vi "Robot Global Data.vi"() -> ()   [LabVIEW 2011]
doc: "This global VI can contain as many global variables as you need. Place a control on the panel, give it a good name. To read or write to it from a VI, drag the icon to the diagram of that VI. You can also drag from the project. Click on the node to change which global you access. You shouldn't have multiple locations writing to a global or it will cause a race-condition."
uses:
  <vilib>/Rock Robotics/WPI/Camera/WPI_CameraImageSize.ctl
  <vilib>/Rock Robotics/WPI/Camera/WPI_CameraWhite Balance Values.ctl
  <vilib>/Rock Robotics/WPI/Camera/WPI_CameraExposure Values.ctl
panel:
  out "Right Drive Distance":dbl
  in  "Binary Path":path
  in  "Harvester Speed":dbl=0.8
  out "Shoot":bool
  out "Shooter Primed":bool
  in  "Right Limit":dbl=3.55
  in  "Left Limit":dbl=1.45
  out "Dashboard DI 2":bool
  out "Record Iteration":dbl
  in  "Shooter Array":dbl[][](array[numeric])
  out "Ball S3 Process":bool
  out "Ball S12 Process":bool
  out "SP 3 Triggered":bool
  out "Conveyer Output":dbl
  out "Harvester Output":dbl
  out "Balls in Robot":dbl
  out "SP 2 Triggered":bool
  out "SP 1 Triggered":bool
  out "Ramp Actuator Output":dbl
  in  "RA Up Volt":dbl=3.7
  in  "RA Down Volt":dbl=1.55
  out "Ramp Actuator Case":dbl
  out "Ramp Actuator Activated":bool
  out "Gyro_Rate":dbl
  in  "Home Position":dbl=2.5
  out "REncoderRate":dbl
  out "LEncoderRate":dbl
  out "Manual Overide":bool
  out "Shooter Output":dbl
  out "Distance To Target":dbl
  out "Home Button":bool
  out "Turret Case":dbl
  out "Lock On Lights":dbl
  out "Raw Turret":dbl
  in  "Enable Color":bool
  in  "Brightness":dbl=30.0
  in  "Exposure":T1=enum."Flicker-free 60 Hz"
  in  "White Balance":T2=enum."Fixed fluorescent 1"
  out "file_read_test_5":dbl
  out "file_read_test_4":dbl
  out "file_read_test_3":dbl
  out "file_read_test_2":dbl
  out "file_read_test_1":dbl
  in  "GlobalVariableArray 2":cluster{"name":string, "va;":dbl}[](array[cluster])=[{"name"="Val1", "va;"=1.0}, {"name"="Val2", "va;"=2.0}, {"name"="Val3", "va;"=3.0}, {"name"="Val4", "va;"=4.0}]
  out "YStart":dbl
  out "XStart":dbl
  in  "Auton Files":string[](array[string])
  in  "Current Auton File":string
  out "Number of Auton Files":dbl
  out "Auton Distance Traveled":dbl
  out "Auton Index":sgl
  out "Robot Angle":dbl
  out "Left Drive Distance":dbl
  in  "Auton Array":dbl[][](array[numeric])
  out "Target Array":T3(array[cluster])
  out "Turret Rotation":dbl
  in  "Camera Settings":T5={"fps"=15, "compression"=30, "Image Size"=enum."320x240"}
  in  "RightShifter_Pos":dbl=0.25
  in  "LeftShifter_Pos":dbl=0.75
  out "Dashboard DI 4":bool
  out "Right Drive Output":dbl
  out "Left Drive Output":dbl
  in  "Camera Address":string="10.0.27.11"
  in  "LED toggle rate (ms)":u32=20
  in  "Enable Vision":bool=TRUE
  # "Sensor Feedback"
  # "Auton and Shooter CSV info"
  # "Motor Outputs"
  # "Ramp Actuator"
  # "Ball Sequencing"
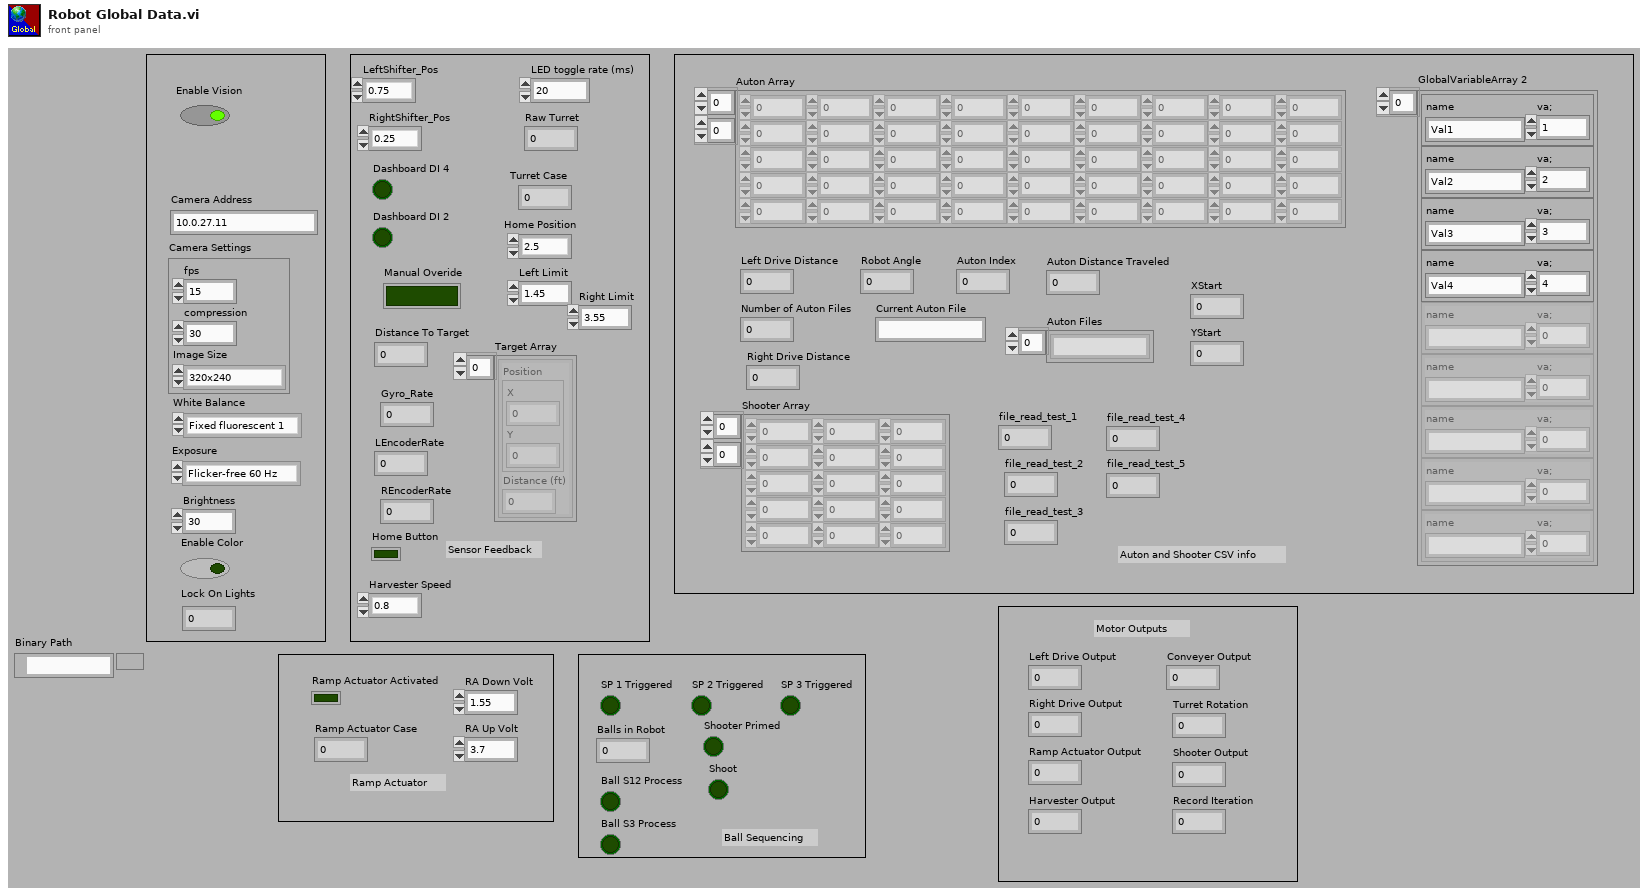
[diagram p1: front panel]
types:
  T1 = typedef "WPI_CameraExposure Values.ctl" = enum16{"Auto", "Flicker-free 50 Hz", "Flicker-free 60 Hz", "Hold current"}
  T2 = typedef "WPI_CameraWhite Balance Values.ctl" = enum16{"Auto", "Fixed indoor", "Fixed outdoor 1", "Fixed outdoor 2", "Fixed fluorescent 1", "Fixed fluorescent 2", "Hold current"}
  T3 = cluster{"Position":cluster{"X":dbl, "Y":dbl}, "Distance (ft)":dbl}[]
  T4 = typedef "WPI_CameraImageSize.ctl" = enum16{"640x480", "320x240", "160x120"}
  T5 = cluster{"fps":i32, "compression":i32, "Image Size":T4}
diagram:
